vi "Initialize SLSC Switch Custom Device.vi"(8 "error in (no error)":errorcluster, 11 "SLSC Custom Device Ref in":T1 format="%.0x") -> (0 "error out":errorcluster, 2 "Endpoint Configuration Section Ref":T1 format="%.0x", 3 "SLSC Custom Device  Ref out":T1 format="%.0x")   [LabVIEW 2017, in "Switch Scripting.lvlib"]
uses:
  Switch Scripting.lvlib
  <vilib>/NI Veristand/Custom Device API/Custom Device Item Ref.ctl
  Scripting Constants.vi
  <vilib>/NI VeriStand/Custom Device API/Custom Device API.lvlib
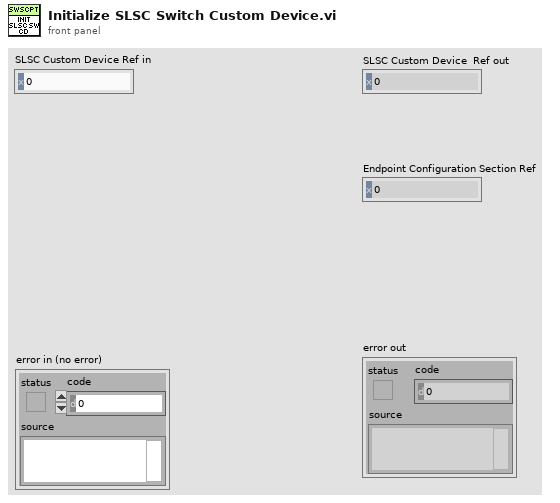
[diagram p1: front panel]
types:
  T1 = typedef "Custom Device API.lvlib/Custom Device Item Ref.ctl" = u64
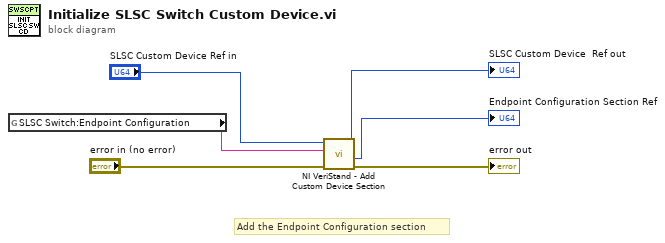
[diagram p0: block diagram]
diagram:
  # "Add the Endpoint Configuration section"
  n1 = global read "Scripting Constants.vi" "SLSC Switch:Endpoint Configuration"() -> (w2:string)
  n2 = call <vilib>:"NI VeriStand - Add Custom Device Section.vi"("error in (no error)"="error in (no error)", "Section Name"=w2, "Parent Ref in"="SLSC Custom Device Ref in") -> ("error out"=→"error out":errorcluster, "Section Ptr"=→"Endpoint Configuration Section Ref":T1, "Parent Ref out"=→"SLSC Custom Device  Ref out":T1)  [unwired: 5 in, 1 out]
